vi "cộng.vi"() -> ()   [LabVIEW 2020]
panel:
  out "Numeric 3":dbl
  in  "Numeric 2":dbl
  in  "Numeric":dbl
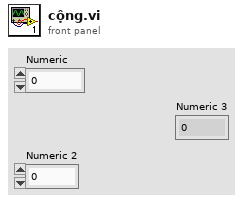
[diagram p1: front panel]
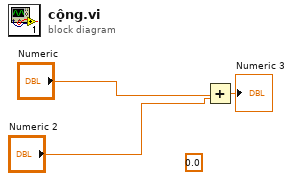
[diagram p0: block diagram]
diagram:
  (unwired) 0.0 ("Numeric 2")
  n1 = Add(x="Numeric", y="Numeric 2") -> ()  [unwired: 1 out]
  "Numeric 3" <- "Numeric"
